vi "modify 3 servo.vi"() -> ()   [LabVIEW 2012]
uses:
  <vilib>/Platform/TimedLoop/XDataNode/timing_clust.ctl
  <vilib>/Platform/TimedLoop/XDataNode/nitl_modes.ctl
  <vilib>/Platform/TimedLoop/XDataNode/wakeup.ctl
  <vilib>/Motion/FlexMotion/FunctionsVIs/AxisResourceConfig.llb/Enable Axes (8 axes).flx
  <vilib>/Motion/FlexMotion/FunctionsVIs/Trajectory.llb/Load Accel/Decel in RPS/sec.flx
  <vilib>/Motion/FlexMotion/FunctionsVIs/StartStopMotion.llb/Start Motion (8 axes).flx
  <vilib>/Motion/FlexMotion/FunctionsVIs/Trajectory.llb/Check Move Complete Status (8 axes).flx
  <vilib>/Motion/FlexMotion/FunctionsVIs/StartStopMotion.llb/Stop Motion (8 axes).flx
  <vilib>/platform/TimedLoop/XDataNode/XDataNode.xnode
  <vilib>/Platform/TimedLoop/XDataNode/XDNodeRunTimeDep.lvlib
panel:
  out "XY Graph":cluster{"Array out":dbl[], "Array out":dbl[]}(graph)={"Array out"=[150.0, 550.0, 750.0, 1150.0, 1550.0, 1950.0, 2350.0, 2750.0, 3150.0, 3550.0, 3950.0, 4350.0, 4750.0, 5150.0, 5550.0, 5950.0, 6350.0, 6750.0, 7150.0, 7550.0, 7950.0, 8350.0, 8750.0, 9150.0, 9550.0, 9950.0, 10350.0, 10750.0, 11150.0, 11550.0, 11950.0, 12350.0, 12750.0, 13150.0, 13550.0, 13950.0, 14350.0, 14750.0, 15150.0, 15550.0, 15950.0, 16350.0, 16750.0, 17150.0, 17550.0, 17950.0, 18350.0, 18750.0, 19150.0, 19550.0, 19950.0, 20350.0, 20750.0, 21150.0, 21550.0, 21950.0, 22350.0, 22750.0, 23150.0, 23550.0, 23950.0, 24350.0, 24750.0, 25150.0, 25550.0, 25950.0, 26350.0, 26750.0, 27150.0, 27550.0, 27950.0, 28350.0, 28750.0, 29150.0, 29550.0, 29950.0, 30350.0, 30750.0, 31150.0, 31550.0, 31950.0, 32350.0, 32750.0, 33150.0, 33550.0, 33950.0, 34350.0, 34750.0, 35150.0, 35550.0, 35950.0, 36350.0, 36750.0, 37150.0, 37550.0, 37950.0, 38350.0, 38750.0, 39150.0, 39550.0, 39950.0, 40350.0, 40750.0, 41150.0, 41550.0, 41950.0, 42350.0, 42750.0, 43150.0, 43550.0, 43950.0, 44350.0, 44750.0, 45150.0, 45550.0, 45950.0, 46350.0, 46750.0, 47150.0, 47550.0, 47950.0, 48350.0, 48750.0, 49150.0, 49550.0, 49950.0, 50350.0, 50750.0, 51150.0, 51550.0, 51950.0, 52350.0, 52750.0, 53150.0, 53550.0, 53950.0, 54350.0, 54750.0, 55150.0, 55550.0, 55950.0, 56350.0, 56750.0, 57150.0, 57550.0, 57950.0, 58350.0, 58750.0, 59150.0, 59550.0, 59950.0, 60350.0, 60750.0, 61150.0, 61550.0, 61950.0, 62350.0, 62750.0, 63150.0, 63550.0, 63950.0, 64350.0, 64750.0, 65150.0, 65550.0, 65950.0, 66350.0, 66750.0, 67150.0, 67550.0, 67950.0, 68350.0, 68750.0, 69150.0, 69550.0, 69950.0, 70350.0, 70750.0, 71150.0, 71550.0, 71950.0, 72350.0, 72750.0, 73150.0, 73550.0, 73950.0, 74350.0, 74750.0, 75150.0, 75550.0, 75950.0, 76350.0, 76750.0, 77150.0, 77550.0, 77950.0, 78350.0, 78750.0, 79150.0, 79550.0, 79950.0, 80350.0, 80750.0, 81150.0, 81550.0, 81950.0, 82350.0, 82750.0, 83150.0, 83550.0, 83950.0, 84350.0, 84750.0, 85150.0, 85550.0, 85950.0, 86350.0, 86750.0, 87150.0, 87550.0, 88150.0], "Array out"=[0.0, -0.18676229438779648, -0.7786488716124618, -1.6037613075254553, -2.427043699264255, -3.435719344710919, -4.213453194236283, -4.9007814645761725, -5.780599648475, -6.5085555979721414, -7.148732291220819, -7.921667513464995, -8.675830813120825, -9.356980938147451, -10.167683522414023, -10.760596880148638, -11.405236925409948, -12.211130405043189, -12.945037490557176, -13.828631013677956, -14.604999314974105, -15.493971212194616, -16.187596371172045, -17.021125613306047, -17.6612464273433, -18.125819206235764, -18.79918465862064, -19.380716119477967, -20.15948722686542, -21.10522541799309, -21.846236148259578, -22.699819042394004, -23.266388844392083, -23.888429241082378, -24.654543707081896, -25.339214222428346, -26.28131677236263, -27.06813448619561, -27.666723076340652, -28.395779147813162, -29.176097410867612, -29.875729585073973, -30.56794030151286, -31.10882662095983, -31.732749448585317, -32.55769424686412, -33.514451119995115, -34.37616443939209, -35.07672211303711, -35.78499111785889, -36.478843286132815, -37.05316982116699, -37.78759029693604, -38.48859500427246, -39.25710179901123, -39.97263510131836, -40.683083395385744, -41.80580851135254, -42.47792366638184, -43.25905916290283, -44.241974491882324, -44.554004008483886, -45.193262187194826, -46.158854960632326, -46.80833903503418, -47.37562478942871, -48.29634655609131, -49.22019755859375, -49.712325773620606, -50.61606026000977, -51.63099437713623, -51.915754838562016, -52.6678331451416, -53.3310635055542, -53.542733958435065, -54.43629842834473, -55.03040620422364, -55.74996280975342, -56.79345120391846, -57.31273671569824, -58.39712869262695, -58.8279015335083, -59.4107217086792, -60.36273583374023, -60.721703887939455, -61.83900872039795, -62.40813848876954, -63.40306784820557, -64.08708527526856, -64.65766790313721, -65.89701293334961, -66.38344146881104, -67.94766823425293, -68.40341908264159, -69.2498214981079, -69.59727843475342, -69.99139451293945, -70.76174532165528, -71.00247296447755, -71.91235416412354, -72.48818943786621, -73.36264321746826, -74.48486542053223, -75.11093610534668, -75.82451363525391, -76.6136398590088, -77.52542095184327, -78.3148824508667, -79.2780724182129, -79.9915940689087, -80.2265661529541, -81.06335734405519, -81.78280219116212, -82.59277136077881, -83.44582340240478, -84.33910847625732, -84.58531228179932, -85.5978994720459, -86.05420911254883, -86.95023226776124, -87.75371944885254, -88.24109793090821, -89.15936101226806, -89.38824226226807, -90.50426187286376, -91.26651019592285, -91.60547349243164, -92.7057910446167, -92.86493503875732, -93.65149081878663, -94.9716371887207, -95.39967194824219, -96.66315679779053, -97.4656940322876, -97.67457052459717, -98.74935127716066, -99.50187661743165, -99.89230466766358, -100.8724819152832, -101.51676922302246, -101.75190894470215, -102.84881786499024, -103.5754711303711, -104.26982621154785, -105.15556759185792, -106.11836640472413, -106.85423973999023, -107.59229236450196, -108.37024274597168, -108.7203260055542, -109.5007909515381, -110.12742042846679, -111.03869860839845, -111.72539823760987, -112.36080075073242, -113.16238803863526, -113.84903178863526, -114.7371200958252, -115.78435239715577, -116.43730098266602, -117.072759375, -117.91323859405517, -118.30199026794435, -119.01646186523438, -119.83788627319336, -120.22624679260254, -121.19742748718262, -122.03634208831788, -123.12609846954346, -123.82307987365724, -124.5148645111084, -125.1440644317627, -125.544383102417, -126.51181988983154, -127.46673973388673, -127.93975725860597, -128.6834536834717, -129.4264236785889, -129.72878609161376, -130.73287964172363, -131.7213828918457, -132.09230909729004, -133.17256601257324, -133.73409620819092, -134.1291622329712, -135.12258285369873, -135.76049993133546, -136.6234425933838, -137.4407319396973, -138.0998831176758, -138.56664217071534, -139.75306958770753, -140.5510247268677, -141.22816901092528, -142.05328144683838, -142.6235846786499, -143.13471182556154, -140.4132265914917, -130.50193086090087, -94.43391153717042, -58.46502193450928, -25.799934828186036, 0.0, 0.0, 0.0, 0.0, 0.0, 0.0, 0.0, 0.0, 0.0, 0.0, 0.0, 0.0, 0.0, 0.0, 0.0, 0.0, 0.0, 0.0, 0.0]}
  in  "MAV":i32=5 min=1
  in  "SAVP":i32=5 min=1
  out "Waveform Chart 2":dbl(graph)
  out "Waveform Chart":i64(graph)=88600
  in  "RUN":bool
  out "indicated vel":dbl
  in  "STOP":bool
  in  "VELOCITY in RPM":dbl=400.0
  in  "CHANGE DIRECTION":bool
  in  "acceleration(rps/s)":dbl=0.03 format="%.2f"
  in  "CHOOSE AXIS":T1={"AXIS1"=FALSE, "AXIS 2"=TRUE, "AXIS 3"=FALSE, "AXIS 4"=FALSE, "AXIS 5"=FALSE, "AXIS 6"=FALSE, "AXIS 7"=FALSE, "AXIS 8"=FALSE}
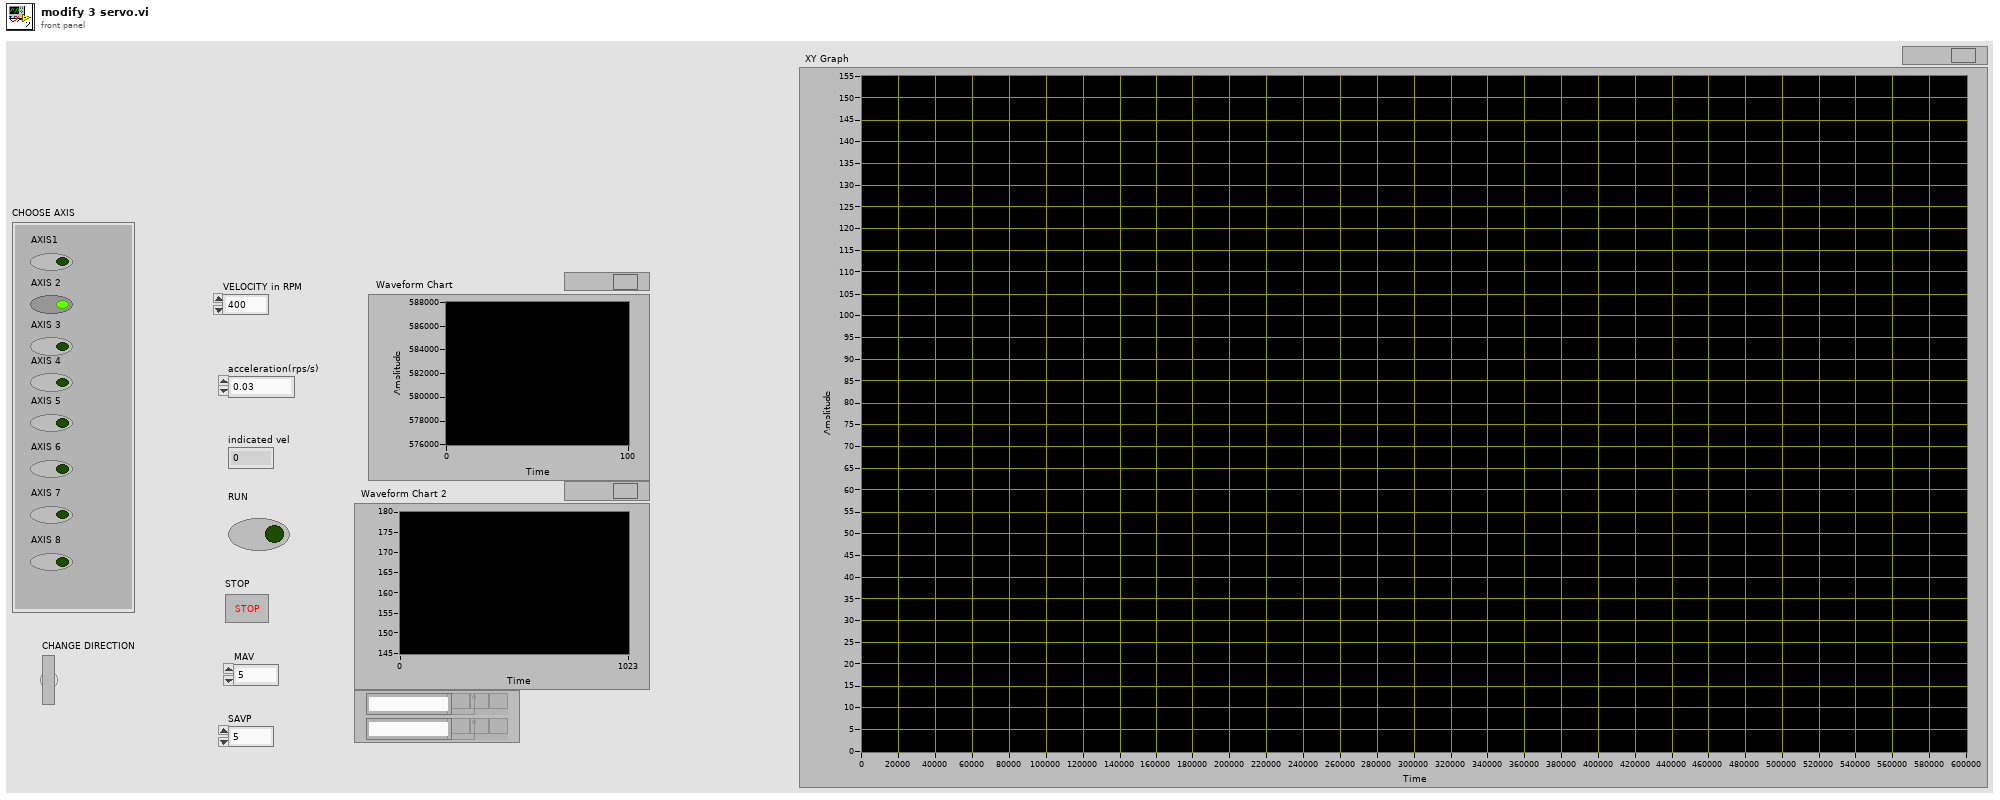
[diagram p1: front panel]
types:
  T1 = cluster{"AXIS1":bool, "AXIS 2":bool, "AXIS 3":bool, "AXIS 4":bool, "AXIS 5":bool, "AXIS 6":bool, "AXIS 7":bool, "AXIS 8":bool}
  T2 = enum16{"Absolute Position", "Relative Position", "Velocity", "Relative to Cap Pos", "Modulus Position", "Absolute Contouring", "Relative Contouring"}
  T3 = typedef "Board Id" = u8
  T4 = typedef "Bd Id Out" = u8
  T5 = typedef "Resource Out (Enum).flx" = u16
  T6 = typedef "XDNodeRunTimeDep.lvlib/timing_clust.ctl" = cluster{"Expected End [f-1]":u64, "Actual End [f-1]":u64, "Finished Late? [f-1]":bool, "Expected End [i-1]":u64, "Actual End [i-1]":u64, "Finished Late? [i-1]":bool, "Expected Start [i]":u64, "Actual Start [i]":u64, "Expected Start [f]":u64, "Actual Start [f]":u64, "Source Name":string, "Structure Name":string, "Period":i64, "Deadline":i64, "Offset":i64, "Start":i64, "Priority":i32, "Timeout":i32, "Mode":T7, "Wakeup Reason":T8, "Error":errorcluster, "Source Type":string, "Secondary Source Type":string, "Global End Time":u64, "Global Start Time":u64, "Frame Duration":u64, "Iteration Duration":u64, "Assigned CPU":i32, "I/O Scan Engine Mode":u32}
  T7 = typedef "XDNodeRunTimeDep.lvlib/nitl_modes.ctl" = enum32{"No Change", "Process missed periods, maintain original phase", "Discard missed periods, maintain original phase", "Process missed periods, ignore original phase", "Discard missed periods, ignore original phase"}
  T8 = typedef "XDNodeRunTimeDep.lvlib/wakeup.ctl" = enum32{"Normal", "Aborted", "Asynchronous wakeup", "Timing source error", "Timed loop error", "Timeout"}
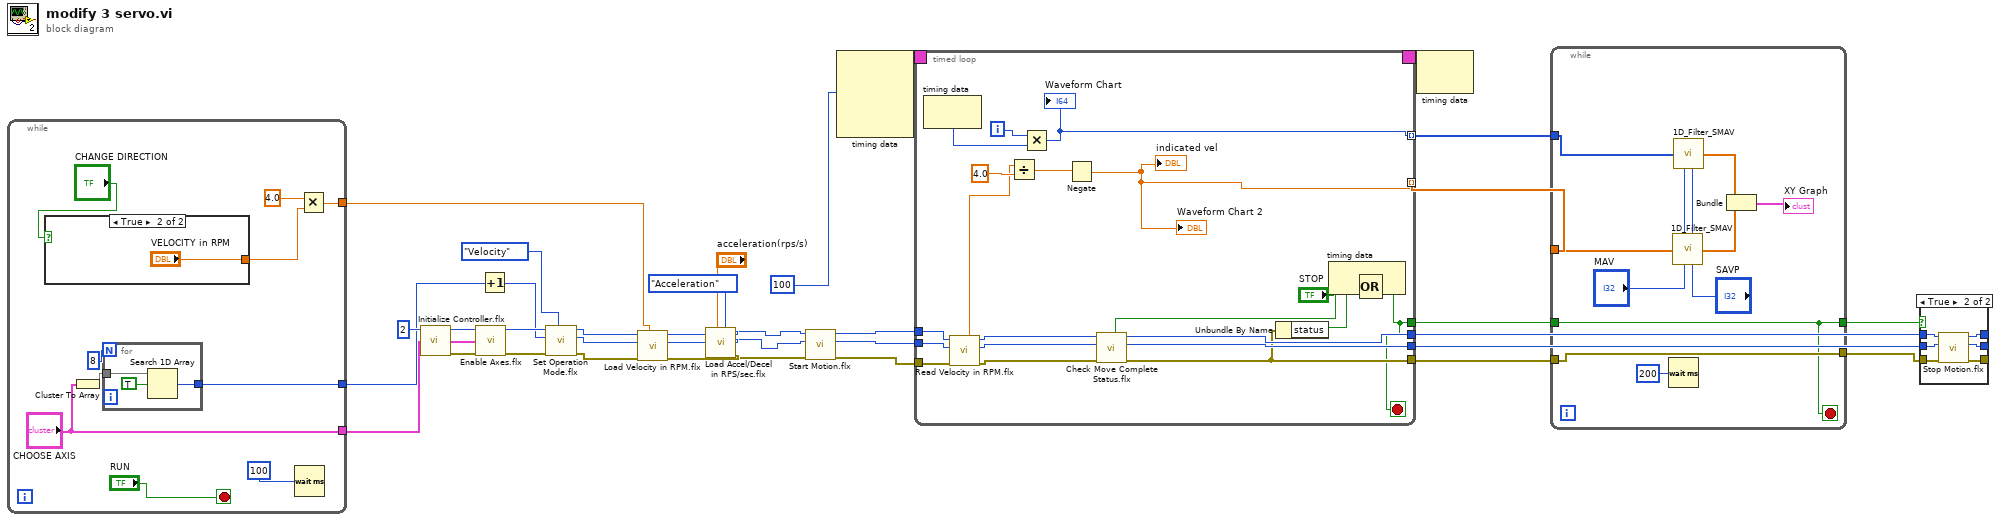
[diagram p0: block diagram]
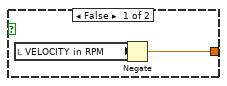
[diagram p2: hidden frame]
diagram:
  n1 = while {
    tunnel: ["CHOOSE AXIS"] -> w29
    tunnel: [w43] -> w28
    tunnel: [w37] -> w10
    stop <- "RUN" stop-if-true
    n2 = case shown="True" "CHANGE DIRECTION" {
      tunnel: [w46 "VELOCITY in RPM"] -> w38
      frame False {
        n3 = local read "VELOCITY in RPM"() -> (w47:dbl)
        n4 = Negate(x=w47) -> (-x=w46:dbl)
      }
      frame True {
      }
    }
    n5 = Cluster To Array(cluster="CHOOSE AXIS") -> (array=w44:bool[])
    n6 = for {
      N: 8 -> [_]
      tunnel: w44 -> [w51]
      tunnel: [w49] -> w43
      n7 = Search 1D Array(1D array=w51, element=TRUE) -> (index of element=w49:i32)  [unwired: 1 in]
    }
    n8 = Wait (ms)(milliseconds to wait=u32 100) -> ()  [unwired: 1 out]
    n9 = Multiply(x=4.0 ("y"), y=w38) -> (x*y=w37:dbl)
  }
  n10 = call <vilib>:"Initialize Controller.flx"("Board ID"=T3 2) -> ("error out"=w33:errorcluster, "Bd ID Out"=w34:T4)  [unwired: 7 in]
  n11 = call-poly <vilib>:"Enable Axes.flx"("Axis Bitmap (Disabled)"=w29, "error in (no error)"=w33, "Board ID"=w34) -> ("error out"=w32:errorcluster, "Bd ID Out"=w31:T4)  [unwired: 5 in]
  n12 = Increment(x=w28) -> (x+1=w27:i32)
  n13 = call <vilib>:"Set Operation Mode.flx"("Position Mode (Absolute)"=T2."Velocity", "error in (no error)"=w32, "Axis or Vector Space"=w27, "Board ID"=w31) -> ("error out"=w12:errorcluster, "Resource Output"=w13:T5, "Bd ID Out"=w14:T4)  [unwired: 2 in]
  n14 = call <vilib>:"Load Velocity in RPM.flx"("Velocity (500)"=w10, "error in (no error)"=w12, "Axis or Vector Space"=w13, "Board ID"=w14) -> ("error out"=w21:errorcluster, "Resource Output"=w22:T5, "Bd ID Out"=w23:T4)  [unwired: 3 in]
  n15 = call "Load Accel/Decel in RPS/sec.flx"("Selector (Both)"=enum16{"Both", "Acceleration", "Deceleration"}."Acceleration", "Value (200)"="acceleration(rps/s)", "error in (no error)"=w21, "Axis or Vector Space"=w22, "Board ID"=w23) -> ("error out"=w15:errorcluster, "Resource Output"=w16:T5, "Bd ID Out"=w17:T4)  [unwired: 2 in]
  n16 = call-poly <vilib>:"Start Motion.flx"("error in (no error)"=w15, "Axis or Vector Space"=w16, "Board ID"=w17) -> ("error out"=w20:errorcluster, "Resource Output"=w19:T5, "Bd ID Out"=w18:T4)  [unwired: 3 in]
  n17 = node-c288(i64 100 ("Period")) -> (w9:T6)  [unwired: 3 in]
  n18 = timed-loop {
    tunnel: [w71] -> w26
    tunnel: [w70] -> w25
    tunnel: [w69] -> w5
    tunnel: [w58] -> w2
    tunnel: w20 -> [w61]
    tunnel: w19 -> [w60]
    tunnel: w18 -> [w59]
    timing: w9 -> [_]
    timing-out: [_] -> w8
    tunnel: [w52] -> w6 mode=indexing
    tunnel: [w54] -> w1 mode=indexing
    i -> [w56]
    stop <- w58 stop-if-true
    n19 = node-c288() -> (w55:i64)  [unwired: 1 in]
    n20 = call <vilib>:"Read Velocity in RPM.flx"("error in (no error)"=w61, "Axis or Vector Space"=w60, "Board ID"=w59) -> ("error out"=w66:errorcluster, "Resource Output"=w67:T5, "Bd ID Out"=w68:T4, "Filtered Velocity"=w57:dbl)  [unwired: 3 in]
    n21 = Divide(x=w57, y=4.0) -> (x/y=w53:dbl)
    n22 = Multiply(x=w56, y=w55) -> (x*y=w54:i64)
    "Waveform Chart" <- w54
    n23 = Negate(x=w53) -> (-x=w52:dbl)
    "indicated vel" <- w52
    "Waveform Chart 2" <- w52
    n24 = call-poly <vilib>:"Check Move Complete Status.flx"("error in (no error)"=w66, "Axis or Vector Space"=w67, "Board ID"=w68) -> ("error out"=w69:errorcluster, "Resource Output"=w70:T5, "Bd ID Out"=w71:T4, "Move Complete"=w64:bool)  [unwired: 3 in]
    n25 = Unbundle By Name(w69) -> ("status"=w65:bool)
    n26 = node-c288() -> ()  [unwired: 1 in, 1 out]
    n27 = Compound Arithmetic op=OR(w65, "STOP", w64) -> (w58:bool)
  }
  n28 = node-c288(w8) -> ()  [unwired: 1 out]
  n29 = while {
    tunnel: w6 -> [w78]
    tunnel: w5 -> [w77]
    tunnel: [w77] -> w4
    tunnel: [w76] -> w3
    tunnel: w2 -> [w76]
    tunnel: w1 -> [w75]
    stop <- w76 stop-if-true
    n30 = Wait (ms)(milliseconds to wait=u32 200) -> ()  [unwired: 1 out]
    n31 = call "1D_Filter_SMAV.vi"("Array in"=w78, "MAV"="MAV", "SAVP"="SAVP") -> ("Array out"=w82:dbl[])
    n32 = call "1D_Filter_SMAV.vi"("Array in"=w75, "MAV"="MAV", "SAVP"="SAVP") -> ("Array out"=w83:dbl[])
    n33 = Bundle("Array out"=w83, "Array out"=w82) -> (→"XY Graph":cluster{"Array out":dbl[], "Array out":dbl[]})  [unwired: 1 in]
  }
  n34 = case shown="True" w3 {
    tunnel: [w85 w93] -> _
    tunnel: [w87 w92] -> _
    tunnel: [w86 w91] -> _
    tunnel: w26 -> [w87 w90]
    tunnel: w25 -> [w86 w89]
    tunnel: w4 -> [w85 w88]
    frame False {
    }
    frame True {
      n35 = call-poly <vilib>:"Stop Motion.flx"("error in (no error)"=w88, "Axis or Vector Space"=w89, "Board ID"=w90) -> ("error out"=w93:errorcluster, "Resource Output"=w91:T5, "Bd ID Out"=w92:T4)  [unwired: 4 in]
    }
  }
